vi "OAT FIR Preprocess Filter (1 Channel).vi"(0 "scaled signal [EU]":waveform(dbl)={"t0"=timestamp(0 s since 1904-01-01), "dt"=0.0, "Y"=[]}, 1 "filter type":T3(ring), 2 "reset? (F)":bool, 7 "freq specs [Hz]":T2={"fpass 1"=100.0, "fstop 1"=200.0, "fpass 2"=0.0, "fstop 2"=0.0} {"fstop 2" format="%#.2f"; "fpass 2" format="%#.3f"; "fstop 1" format="%#.2f"; "fpass 1" format="%#.3f"}, 9 "ripple specs [dB]":T1={"passband ripple"=0.1, "stopband attenuation"=60.0} {"stopband attenuation" format="%#.2f"; "passband ripple" format="%#.2f"}, 11 "error in (no error)":errorcluster) -> (4 "filtered scaled signal [EU]":waveform(dbl), 8 "taps":i32, 15 "error out":errorcluster)   [LabVIEW 2017, in "SoundVib_RefDataProcess.lvlib"]
doc: "Designs an FIR filter and filters the <B>scaled signal [EU]</B>. Wire data to the <B>scaled signal [EU]</B> input to determine the polymorphic instance to use or manually select the instance."
uses:
  <vilib>/addons/Sound and Vibration/Order Analysis/Referece Data Processing/SoundVib_RefDataProcess.lvlib
  <vilib>/addons/_NISVFA/_Shared subVIs/Common/svc_Check for Waveform Parameter Continuity (no state).vi
  <vilib>/addons/_NISVFA/_Shared subVIs/Common/svc_Get SV Channel Info.vi
  <vilib>/measure/macond.llb/Continuous Waveform Convolution for 1 Chan.vi
  <vilib>/addons/_NISVFA/_Shared subVIs/Common/svc_Engineering Units to Unit Label.vi
  <vilib>/addons/_NISVFA/_Shared subVIs/Common/svc_Unit Label to Engineering Units.vi
  <vilib>/measure/NI_MAPro.lvlib
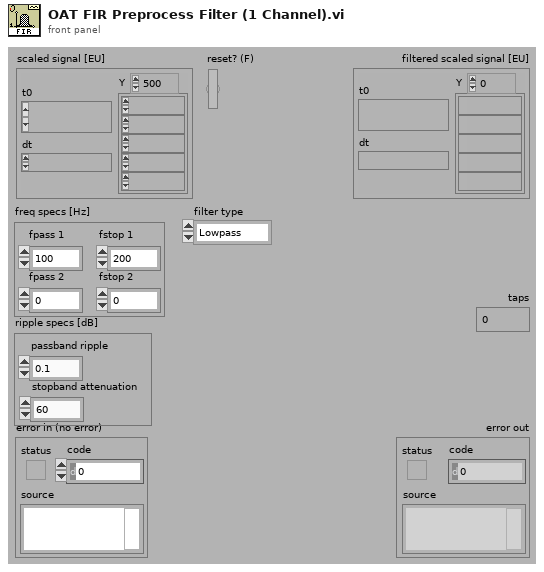
[diagram p1: front panel]
types:
  T1 = cluster{"passband ripple":dbl, "stopband attenuation":dbl}
  T2 = cluster{"fpass 1":dbl, "fstop 1":dbl, "fpass 2":dbl, "fstop 2":dbl}
  T3 = enum32{"Lowpass", "Highpass", "Bandpass", "Bandstop"}
  T4 = cluster{"dt":bool, "t0 continuity":bool, "array length":bool, "channel info":bool, "name":bool}
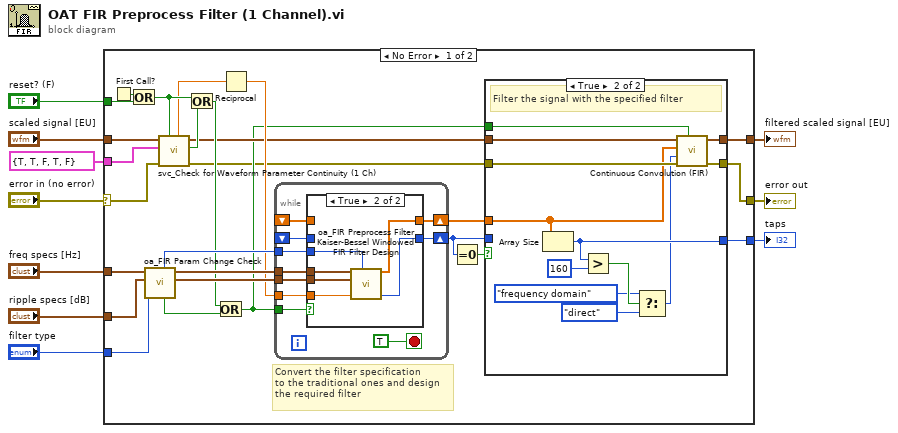
[diagram p0: block diagram]
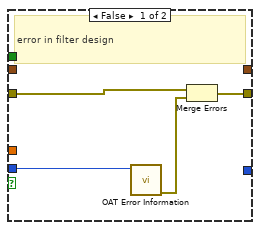
[diagram p3: hidden frame]
diagram:
  n1 = case shown="No Error" "error in (no error)" {
    selector: "error in (no error)" -> [w22 w71]
    tunnel: "filter type" -> [w33 _]
    tunnel: [w14 w71] -> w9
    tunnel: "scaled signal [EU]" -> [w26 _]
    tunnel: [w17 _] -> w8
    tunnel: "freq specs [Hz]" -> [w35 _]
    tunnel: "ripple specs [dB]" -> [w34 _]
    tunnel: [w13 _] -> w5
    tunnel: "reset? (F)" -> [w21 _]
    tunnel: T4 {"dt"=TRUE, "t0 continuity"=TRUE, "array length"=FALSE, "channel info"=TRUE, "name"=FALSE} ("checks for channel parameter change") -> [w12 _]
    frame No Error {
      # "Convert the filter specification\nto the traditional ones and design\nthe required filter"
      n2 = First Call?() -> (First Call?: T/F=w27:bool)
      n3 = Or(x=w27, y=w21) -> (x .or. y?=w24:bool)
      n4 = call <vilib>:"oa_FIR Param Change Check.vi"("filter type in"=w33, "ripple specs in [dB]"=w34, "freq specs in [Hz]"=w35) -> ("ripple specs out [dB]"=w31:cluster{"pass band":dbl, "stop band":dbl}, "freq specs out [Hz]"=w32:T2, "chang?"=w29:bool, "filter type out"=w30:T3)  [unwired: 4 in, 1 out]
      n5 = call <vilib>:"svc_Check for Waveform Parameter Continuity (1 Ch).vi"("restart averaging (F)"=w24, "error in (no error)"=w22, "checks for channel parameter change"=w12, "scaled signal [EU]"=w26) -> ("error out"=w15:errorcluster, "waveform parameter changed"=w25:bool, "dup scaled signal [EU]"=w18:waveform(dbl), "dt"=w19:dbl)  [unwired: 2 in, 2 out]
      n6 = Or(x=w24, y=w25) -> (x .or. y?=w23:bool)
      n7 = Or(x=w23, y=w29) -> (x .or. y?=w16:bool)
      n8 = Reciprocal(x=w19) -> (1/x=w20:dbl)
      n9 = while {
        shift-right: [w45] -> w28
        shift-left: _ -> [w42]
        tunnel: w16 -> [w43]
        shift-right: [w46] -> w11
        shift-left: _ -> [w41]
        tunnel: w32 -> [w40]
        tunnel: w31 -> [w39]
        tunnel: w30 -> [w38]
        tunnel: w20 -> [w37]
        stop <- TRUE stop-if-true
        n10 = case shown="True" w43 {
          tunnel: [w47 w50] -> w46
          tunnel: [w48 w51] -> w45
          tunnel: w42 -> [w48 _]
          tunnel: w41 -> [w47 _]
          tunnel: w40 -> [_ w54]
          tunnel: w39 -> [_ w53]
          tunnel: w38 -> [_ w49]
          tunnel: w37 -> [_ w52]
          frame False {
          }
          frame True {
            n11 = call <vilib>:"oa_FIR Preprocess Filter Kaiser-Bessel Windowed FIR Filter Design.vi"("filter types"=w49, "fs [Hz]"=w52, "ripple specs [dB]"=w53, "freq specs [Hz]"=w54) -> ("error"=w50:i32, "FIR Windowed Coefficients"=w51:dbl[])  [unwired: 6 in]
          }
        }
      }
      n12 = Equal To 0?(x=w11) -> (x = 0?=w36:bool)
      n13 = case shown="True" w36 {
        tunnel: w28 -> [_ w65]
        tunnel: w18 -> [_ w70]
        tunnel: [_ w69] -> w17
        tunnel: w16 -> [_ w68]
        tunnel: w15 -> [w56 w67]
        tunnel: [w55 w66] -> w14
        tunnel: [_ w64] -> w13
        tunnel: w11 -> [w57 _]
        frame False {
          # "error in filter design"
          n14 = call <vilib>:"OAT Error Information.vi"("error code"=w57) -> ("error out"=w58:errorcluster)  [unwired: 6 in]
          n15 = Merge Errors(w56, w58) -> (w55:errorcluster)
        }
        frame True {
          # "Filter the signal with the specified filter"
          n16 = Array Size(array=w65) -> (size(s)=w64:i32)
          n17 = Greater?(x=w64, y=160) -> (0:w62:bool)
          n18 = Select(t=enum32{"direct", "frequency domain"}."frequency domain" ("algorithm"), s=w62, f=enum32{"direct", "frequency domain"}."direct" ("algorithm")) -> (s? t:f=w59:enum32{"direct", "frequency domain"})
          n19 = call-poly <vilib>:"Continuous Convolution (FIR).vi"("reset"=w68, "error in (no error)"=w67, "algorithm"=w59, "kernel"=w65, "signal in"=w70) -> ("error out"=w66:errorcluster, "signal out"=w69:waveform(dbl))  [unwired: 5 in]
        }
      }
    }
    frame Error {
    }
  }
  "error out" <- w9
  "filtered scaled signal [EU]" <- w8
  "taps" <- w5
